vi "IECMemory.SetStatus.vi"(0 "i ref in":refnum<vi>, 2 "MemoryStatusBits":T1=[FALSE, FALSE, FALSE, FALSE, FALSE, FALSE, FALSE, FALSE, FALSE, FALSE, FALSE, FALSE, FALSE], 3 "ms timeout (100)":i32=100, 5 "error in (no error)":errorcluster) -> (14 "i ref out":refnum<vi>, 17 "timed out":bool, 19 "error out":errorcluster)   [LabVIEW 2014, in "IECMemory.lvlib"]
uses:
  IECMemory.lvlib
  CS_Core/CSSystem/CoreDefs/CoreDefs.error_type.ctl
  CS_Core/CSSystem/CoreLib/CoreLib.lvlib
  instr.lib/GPIB_Memory/Memory_Status.ctl
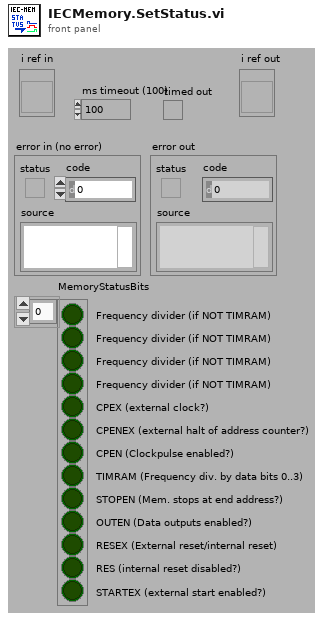
[diagram p1: front panel]
types:
  T1 = typedef "IECMemoryDriver.lvlib/Memory_Status.ctl" = bool[]
  T2 = typedef "CoreDefs.error_type.ctl" = enum16{"no error", "can't load process", "can't unload process", "process does not exist", "can't install process", "can't remove process", "unknown function", "time out", "can't execute function", "duplicate queue name", "super not found", "caller queue invalid", "can't ping process", "unknown error", "VISA Error", "VISA timeout", "GPIB timeout", "GPIB error", "communication error", "data type mismatch", "can't read data from OPC server", "can't write data to OPC server", "OET error", "function not implemented", "process already exists", "invalid Shared Variable name", "error writing Shared Variable", "error reading Shared Variable", "invalid client name", "corrupt database", "unknown class", "call not authorized", "parameter out of range", "OET timeout: can't get data to modify", "invalid queue name", "requested operation incompatible with current state", "event undefined", "event disabled", "state undefined", "caller is not a friend", "EventBuilder: bad eventID", "EventBuilder: no DAQ devices", "a thread must not stop itself", "UNUSED ELEMENT4", "DiscArchiver: eventData incomplete", "DiscArchiver: eventData does not belong to run", "DiscArchiver: can't open file", "DiscArchiver: can't write to file", "DiscArchiver: available disc space low", "can't acquire semaphore", "error reading data from database", "notifier object is not existing", "can't register process", "can't unregister process", "illegal event type", "object disabled", "object already exists", "can't change state", "Instrument not found", "no connection to remote node", "invalid reference", "N/A", "UNUSED ELEMENT 1", "element not found", "illegal TCP/IP connection detected", "object does not exist", "invalid access ID", "unknown CS system", "invalid privilige", "unsupported data type", "unsupported server type", "IO server already exists", "Shared Variable already exists"}
  T3 = typedef "IECMemory.lvlib/IECMemory.i attribute.ctl" = cluster{"EndAddress":u32, "MemoryStatusBits":T1, "IEC Finished":bool, "Call Process":string, "Call Event":string}
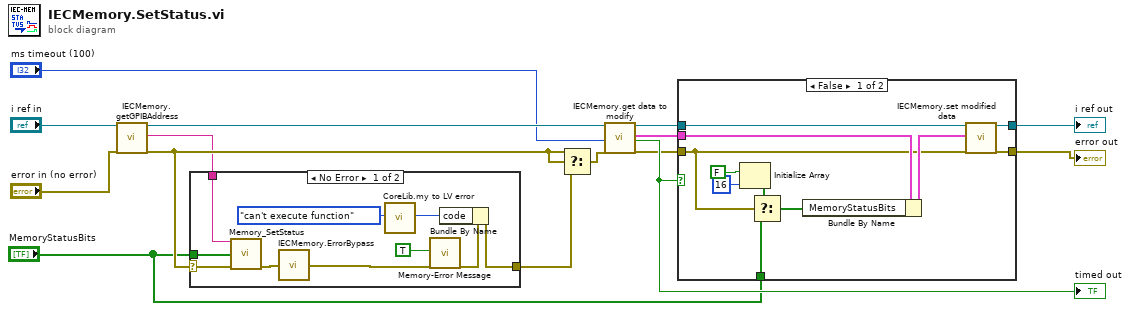
[diagram p0: block diagram]
diagram:
  n1 = call "IECMemory.getGPIBAddress.vi"("i ref in"="i ref in", "error in (no error)"="error in (no error)") -> ("i ref out"=w10:refnum<vi>, "GPIBAddress"=w1:string, "error out"=w12:errorcluster)  [unwired: 14 in, 1 out]
  n2 = case shown="No Error" w12 {
    selector: w12 -> [w19 w26]
    tunnel: [w21 w26] -> w13
    tunnel: "MemoryStatusBits" -> [w18 _]
    tunnel: w1 -> [w17 _]
    frame No Error {
      n3 = call "Memory_SetStatus.vi"("address string"=w17, "MemoryStatus"=w18, "error in"=w19) -> ("error out"=w25:errorcluster)  [unwired: 11 in, 1 out]
      n4 = call "IECMemory.ErrorBypass.vi"("error in (no error)"=w25) -> ("error out"=w16:errorcluster)  [unwired: 14 in]
      n5 = call "CoreLib.my to LV error.vi"("ErrorTypes"=CoreDefs.error_type."can't execute function") -> ("LV error code"=w20:i32)  [unwired: 17 in, 1 out]
      n6 = call "Memory-Error Message.vi"("add message to source"=TRUE, "error in (no error)"=w16) -> ("error out"=w22:errorcluster)  [unwired: 14 in, 3 out]
      n7 = Bundle By Name(cluster=w22, "code"=w20) -> (w21:errorcluster)
    }
    frame Error {
    }
  }
  n8 = Select(t=w12, s=w12, f=w13) -> (s? t:f=w11:errorcluster)
  n9 = call "IECMemory.get data to modify.vi"("i ref in"=w10, "ms timeout (10000)"="ms timeout (100)", "error in (no error)"=w11) -> ("i ref out"=w7:refnum<vi>, "i attribute"=w3:T3, "timed out"=w8:bool, "error out"=w5:errorcluster)  [unwired: 13 in]
  "timed out" <- w8
  n10 = case shown="False" w8 {
    tunnel: w7 -> [w30 w39]
    tunnel: [w32 w39] -> w6
    tunnel: [w31 w38] -> w4
    tunnel: w5 -> [w28 w38]
    tunnel: w3 -> [w37 _]
    tunnel: "MemoryStatusBits" -> [w36 _]
    frame False {
      n11 = Initialize Array(FALSE, 16 ("dimension size")) -> (w34:bool[])
      n12 = Select(t=w34, s=w28, f=w36) -> (s? t:f=w33:T1)
      n13 = Bundle By Name(cluster=w37, "MemoryStatusBits"=w33) -> (w29:T3)
      n14 = call "IECMemory.set modified data.vi"("i ref in"=w30, "i attribute"=w29, "error in (no error)"=w28) -> ("i ref out"=w32:refnum<vi>, "error out"=w31:errorcluster)  [unwired: 15 in]
    }
    frame True {
    }
  }
  "error out" <- w4
  "i ref out" <- w6
